vi "niScope Configure Trigger Width.vi"(0 "instrument handle":refnum<k15>, 1 "polarity":T1=1 items=["Positive"=1, "Negative"=2, "Either"=3], 2 "trigger coupling":T3=1 items=["AC"=0, "DC"=1, "HF Reject"=3, "LF Reject"=4, "AC Plus HF Reject"=1001], 3 "width low threshold":dbl caption="low threshold" format="%^.3e", 5 "trigger source":T2="0", 7 "trigger level":dbl format="%.2f", 9 "width condition":i32(ring)=1 items=["Within"=1, "Outside"=2], 11 "error in":errorcluster, 12 "trigger holdoff":dbl format="%.4f", 13 "trigger delay":dbl format="%.4f", 14 "width high threshold":dbl caption="high threshold" format="%^.3e") -> (4 "instrument handle out":refnum<k15>, 15 "error out":errorcluster)   [LabVIEW 2020]
doc: "Configures common properties for width triggering."
uses:
  niScope trigger coupling.ctl
  niScope trigger source.ctl
  niScope trigger polarity.ctl
  niScope_32.dll
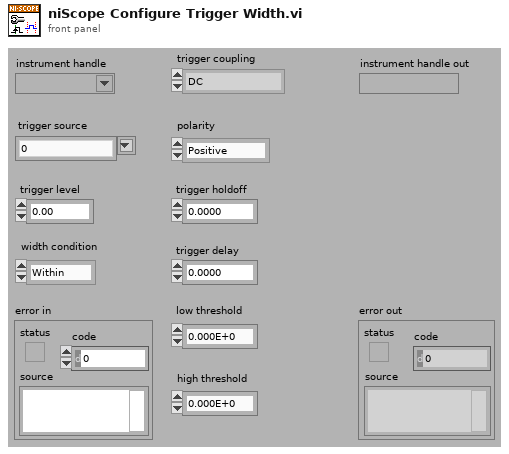
[diagram p1: front panel]
types:
  T1 = typedef "niScope trigger polarity.ctl" = i32
  T2 = typedef "niScope trigger source.ctl" = string
  T3 = typedef "niScope trigger coupling.ctl" = u16
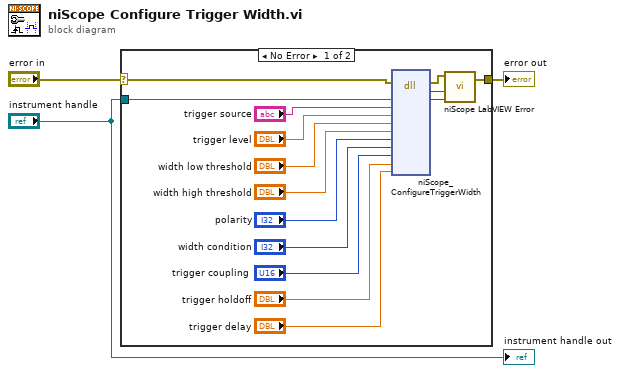
[diagram p0: block diagram]
diagram:
  n1 = case shown="No Error" "error in" {
    selector: "error in" -> [w5 w19]
    tunnel: [w15 w19] -> w3
    tunnel: "instrument handle" -> [w18 _]
    frame No Error {
      n2 = dll-call lib="niScope_*.*" fn="niScope_ConfigureTriggerWidth"(error in=w5, "instrument handle"=w18, "triggerSource"="trigger source", "level"="trigger level", "widthLowThreshold"="width low threshold", "widthHighThreshold"="width high threshold", "widthPolarity"="polarity", "widthCondition"="width condition", "coupling"="trigger coupling", "holdoff"="trigger holdoff", "delay"="trigger delay") -> (error out=w4:errorcluster, "status"=w17:i32, "instrument handle"=w16:u32)  [unwired: 11 in, 1 out]
      n3 = call "niScope LabVIEW Error.vi"("instrument handle"=w16, "niScope error code (0)"=w17, "error in (no error)"=w4) -> ("error out"=w15:errorcluster)  [unwired: 2 in]
    }
    frame Error {
    }
  }
  "error out" <- w3
  "instrument handle out" <- "instrument handle"
